vi "WSVCAP SHL FPGA LL I2C Debug Global.vi"() -> ()   [LabVIEW 2012]
panel:
  out "Boolean array":bool[](array[boolean])
  in  "Socket Mask":u64
  in  "I2C CH (1-32)":i32
  in  "I2C SCL":bool
  in  "I2C SDA":bool
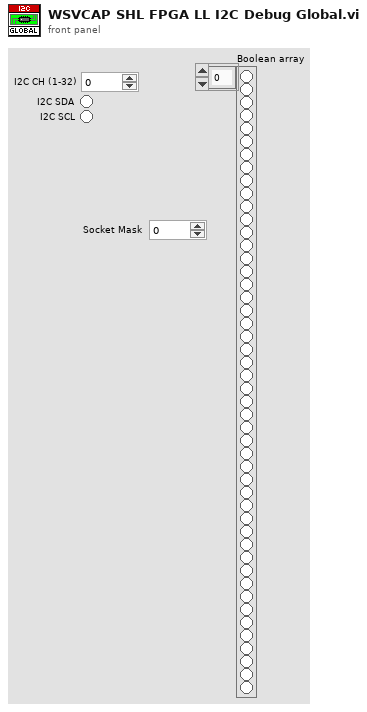
[diagram p1: front panel]
diagram:
